vi "load_Switches.vi"() -> (3 "output array":string[][](array[string]))   [LabVIEW 2017]
doc: "loads the setup data of the Switches"
uses:
  Classes/PrepLineObject/PrepLineObject.lvclass
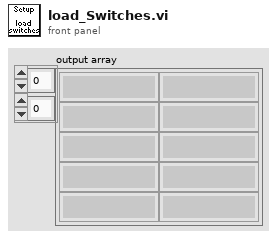
[diagram p1: front panel]
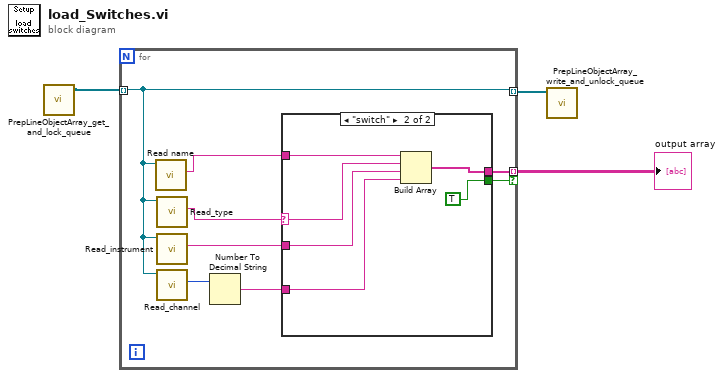
[diagram p0: block diagram]
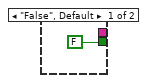
[diagram p2: hidden frame]
diagram:
  n1 = call "PrepLineObjectArray_get_and_lock_queue.vi"() -> ("PrepLineObjects"=w2:refnum<class "PrepLineObject.lvclass">[])  [unwired: 10 in, 1 out]
  n2 = for {
    tunnel: w2 -> [w10] mode=indexing
    tunnel: [w11] -> w3 mode=indexing if=w4
    tunnel: [w10] -> w1 mode=indexing
    n3 = call-dynamic "Read name.vi"("PrepLineObject in"=w10) -> ("name"=w9:string)  [unwired: 8 in, 2 out]
    n4 = call-dynamic "Read_type.vi"("PrepLinePictureObjects in"=w10) -> ("type"=w5:string)  [unwired: 8 in, 2 out]
    n5 = call-dynamic "Read_instrument.vi"("PrepLinePictureObjects in"=w10) -> ("instrument name"=w8:string)  [unwired: 7 in, 2 out]
    n6 = call-dynamic "Read_channel.vi"("PrepLineObject in"=w10) -> ("channel"=w7:u16)  [unwired: 8 in, 2 out]
    n7 = Number To Decimal String(number=w7) -> (decimal integer string=w6:string)  [unwired: 1 in]
    n8 = case shown="\"switch\"" w5 {
      selector: w5 -> [_ w14]
      tunnel: [_ w18] -> w11
      tunnel: w9 -> [_ w17]
      tunnel: w8 -> [_ w16]
      tunnel: w6 -> [_ w15]
      tunnel: [FALSE TRUE] -> w4
      frame "False", Default {
      }
      frame "switch" {
        n9 = Build Array(w17, w14, w16, w15) -> (w18:string[])
      }
    }
  }
  "output array" <- w3
  n10 = call "PrepLineObjectArray_write_and_unlock_queue.vi"("PrepLineObjArray"=w1) -> ()  [unwired: 10 in, 1 out]
